vi "MainUI_Alarms.vi"(8 "error in":errorcluster, 10 "Direcciones IP":string[](array[string])=["192.168.169.1", "192.168.169.2", "192.168.169.3", "192.168.169.4", "192.168.169.5", "192.168.169.6"]) -> (0 "error out":errorcluster, 2 "Descripcion de Alarmas":string)   [LabVIEW 2015]
uses:
  <vilib>/Utility/error.llb/DialogType.ctl
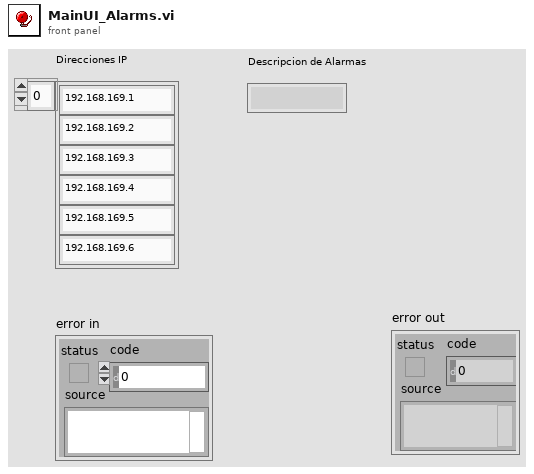
[diagram p1: front panel]
types:
  T1 = typedef "DialogType.ctl" = u16
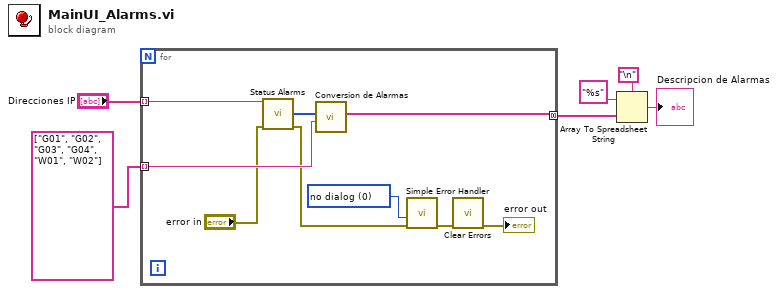
[diagram p0: block diagram]
diagram:
  n1 = for {
    tunnel: string[] ["G01", "G02", "G03", "G04", "W01", "W02"] -> [w14] mode=indexing
    tunnel: [w13] -> w2 mode=concatenating
    tunnel: "Direcciones IP" -> [w12] mode=indexing
    w11 = T1 0 items=["no dialog", "OK message", "continue or stop message", "OK message + warnings", "continue/stop + warnings"] ("type of dialog (OK msg:1)")
    n2 = call "Status Alarms.vi"("error in"="error in", "Network Path In"=w12) -> ("error out"=w10:errorcluster, "Data"=w15:i16[])  [unwired: 7 in, 1 out]
    n3 = call "Conversion de Alarmas.vi"("Fuente"=w14, "Data Alarms"=w15) -> ("Description Alarms"=w13:string[])  [unwired: 9 in]
    n4 = call <vilib>:"Simple Error Handler.vi"("type of dialog (OK msg:1)"=w11, "error in (no error)"=w10) -> ("error out"=w8:errorcluster)  [unwired: 3 in, 4 out]
    n5 = call <vilib>:"Clear Errors.vi"("error in (no error)"=w8) -> ("error out"=→"error out":errorcluster)  [unwired: 5 in, 1 out]
  }
  n6 = Array To Spreadsheet String(delimiter (Tab)="\n", array=w2, 3:"%s" ("format string")) -> (spreadsheet string=→"Descripcion de Alarmas":string)
